vi "From String Array.vi"(8 "error in (no error)":errorcluster, 9 "String Array":string[](array[string]), 11 "Wait On Boolean Config in":refnum<class "Wait On Boolean Step Config.lvclass">) -> (0 "error out":errorcluster, 1 "String Array 2":string[](array[string]), 3 "Wait On Boolean Config out":refnum<class "Wait On Boolean Step Config.lvclass">)   [LabVIEW 2015, in "Wait On Boolean Step Config.lvclass"]
uses:
  Wait On Boolean Step Config.lvclass
  <vilib>/NI/Tag Bus/tag/Data Type.ctl
  <vilib>/NI/Tag Bus Module Framework/channel/channel classification.ctl
  Wait On Boolean Step Config.lvclass/Wait On Boolean Step Config.ctl
  classes/Step/Config/Step Config.lvclass
  <vilib>/NI/Tag Bus Module Framework/channel/TBM channel.lvclass
  <vilib>/NI/Tag Bus/tag/tag descriptor.lvclass
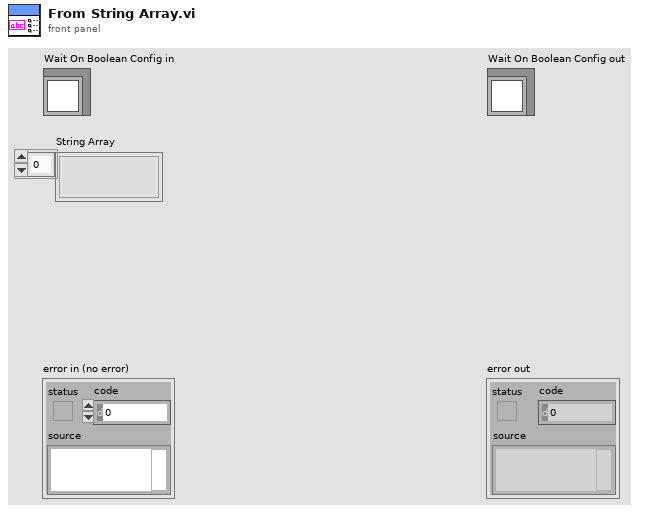
[diagram p1: front panel]
types:
  T1 = typedef "TBM channel.lvclass/channel classification.ctl" = enum16{"input data", "output data", "processing parameter", "processing result"}
  T2 = typedef "tag bus.lvlib/tag descriptor.lvclass/Data Type.ctl" = enum16{"Double", "Single", "I64", "I32", "I16", "I8", "U64", "U32", "U16", "U8", "Boolean", "String", "Array of Double", "Array of Single", "Array of I64", "Array of I32", "Array of I16", "Array of I8", "Array of U64", "Array of U32", "Array of U16", "Array of U8", "Array of Boolean", "Array of String"}
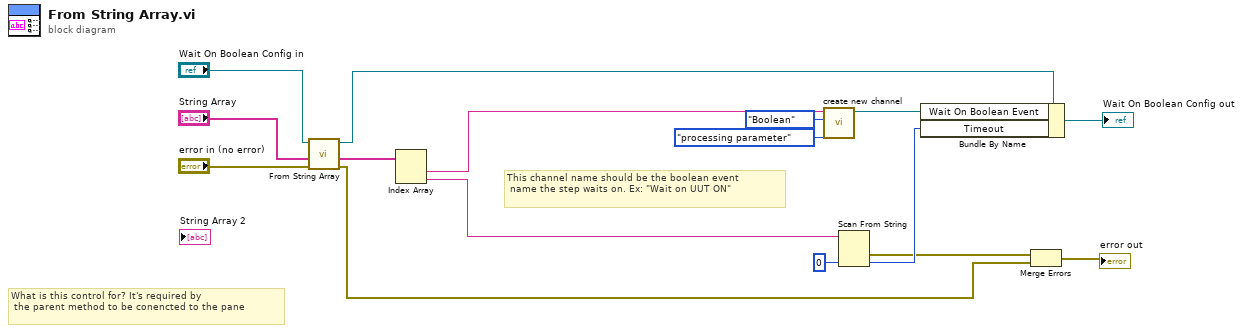
[diagram p0: block diagram]
diagram:
  # "What is this control for? It's required by\n the parent method to be conencted to the pane"
  # "This channel name should be the boolean event\n name the step waits on. Ex: \"Wait on UUT ON\""
  n1 = call-parent "From String Array.vi"("error in (no error)"="error in (no error)", "String Array"="String Array", "Step Config in"="Wait On Boolean Config in") -> ("error out"=w7:errorcluster, "Elements Left 2"=w13:string[], "Step Config out"=w12:refnum<class "Wait On Boolean Step Config.lvclass">)  [unwired: 6 in]
  n2 = Index Array(array=w13) -> (element #1=w6:string, element #2=w11:string)  [unwired: 2 in]
  n3 = call <vilib>:"create new channel.vi"("channel classification"=channel_classification."processing parameter", "data type"=Data_Type."Boolean", "channel name"=w6) -> ("channel"=w3:refnum<class "TBM channel.lvclass">)  [unwired: 8 in]
  n4 = Scan From String(input string=w11, default 1=0 ("Jump Index")) -> (error out=w8:errorcluster, output 1=w9:i32)  [unwired: 3 in, 2 out]
  n5 = Bundle By Name(cluster=w12, "Wait On Boolean Event"=w3, "Timeout"=w9) -> (→"Wait On Boolean Config out":refnum<class "Wait On Boolean Step Config.lvclass">)
  n6 = Merge Errors(w8, w7) -> (→"error out":errorcluster)
